vi "例5.4“数组子集”函数.vi"() -> ()   [LabVIEW 2017]
panel:
  out "子数组":i32[][](array[numeric])
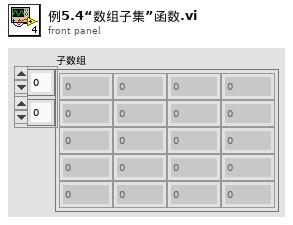
[diagram p1: front panel]
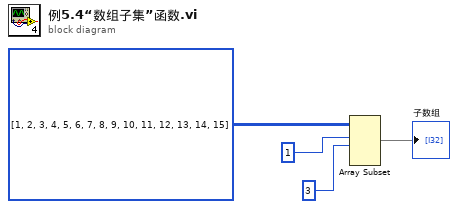
[diagram p0: block diagram]
diagram:
  n1 = Array Subset(array=i32[][] [[1, 2, 3], [4, 5, 6], [7, 8, 9], [10, 11, 12], [13, 14, 15]], index (row)=1 ("索引"), length (row)=3 ("长度")) -> (→"子数组":i32[][])  [unwired: 2 in]
